vi "Interface_Asset_Write Asset.vi"(8 "error in (no error)":errorcluster, 10 "TagBus DVR":refnum<data-value>, 11 "Asset_Interface in":refnum<class "Grid.lvclass">) -> (0 "error out":errorcluster, 2 "TagBus DVR out":refnum<data-value>, 3 "Asset_Interface out":refnum<class "Grid.lvclass">)   [LabVIEW 2015, in "Grid.lvclass"]
uses:
  Grid.lvclass
  TagBus/TagBus.lvclass
  AssetInterface/Interface_Asset.lvclass
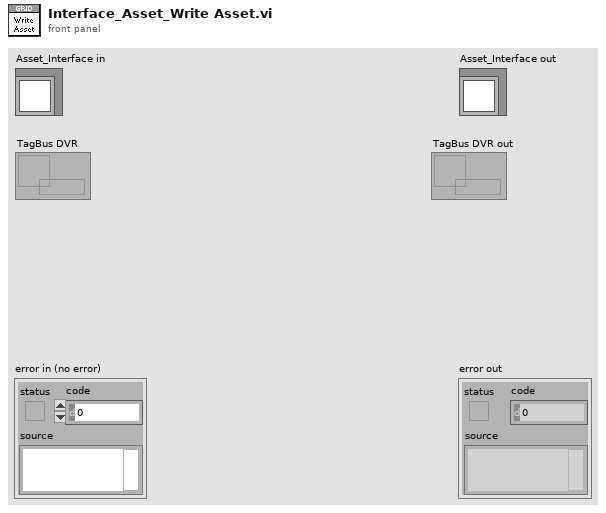
[diagram p1: front panel]
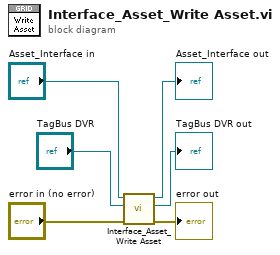
[diagram p0: block diagram]
diagram:
  n1 = call-parent "Interface_Asset_Write Asset.vi"("error in (no error)"="error in (no error)", "TagBus DVR"="TagBus DVR", "Asset_Interface in"="Asset_Interface in") -> ("error out"=→"error out":errorcluster, "TagBus DVR out"=→"TagBus DVR out":refnum<data-value>, "Asset_Interface out"=→"Asset_Interface out":refnum<class "Grid.lvclass">)  [unwired: 6 in]
